vi "readslow.vi"(5 "Write enable":bool, 6 "Iteration number":i32, 7 "string":string, 8 "Slow data time":i32, 9 "mean value input":dbl[](array[numeric]), 10 "data  in":string[](array[string]), 11 "refnum in":refnum<file>) -> (0 "error out":errorcluster, 1 "mean value output":dbl[](array[numeric]), 2 "data out":string[](array[string]), 3 "refnum out":refnum<file>, 4 "Number of errors":bool)   [LabVIEW 2012]
panel:
  in  "array of datanames":string[](array[string])
  in  "number of iterations to\nbuild mean value":i32=5
  out "slow data time":u64
  out "mean value":dbl[](array[numeric])
  out "array of datanames":string[](array[string])
  out "data":string[](array[string])
  in  "Write Enable":bool
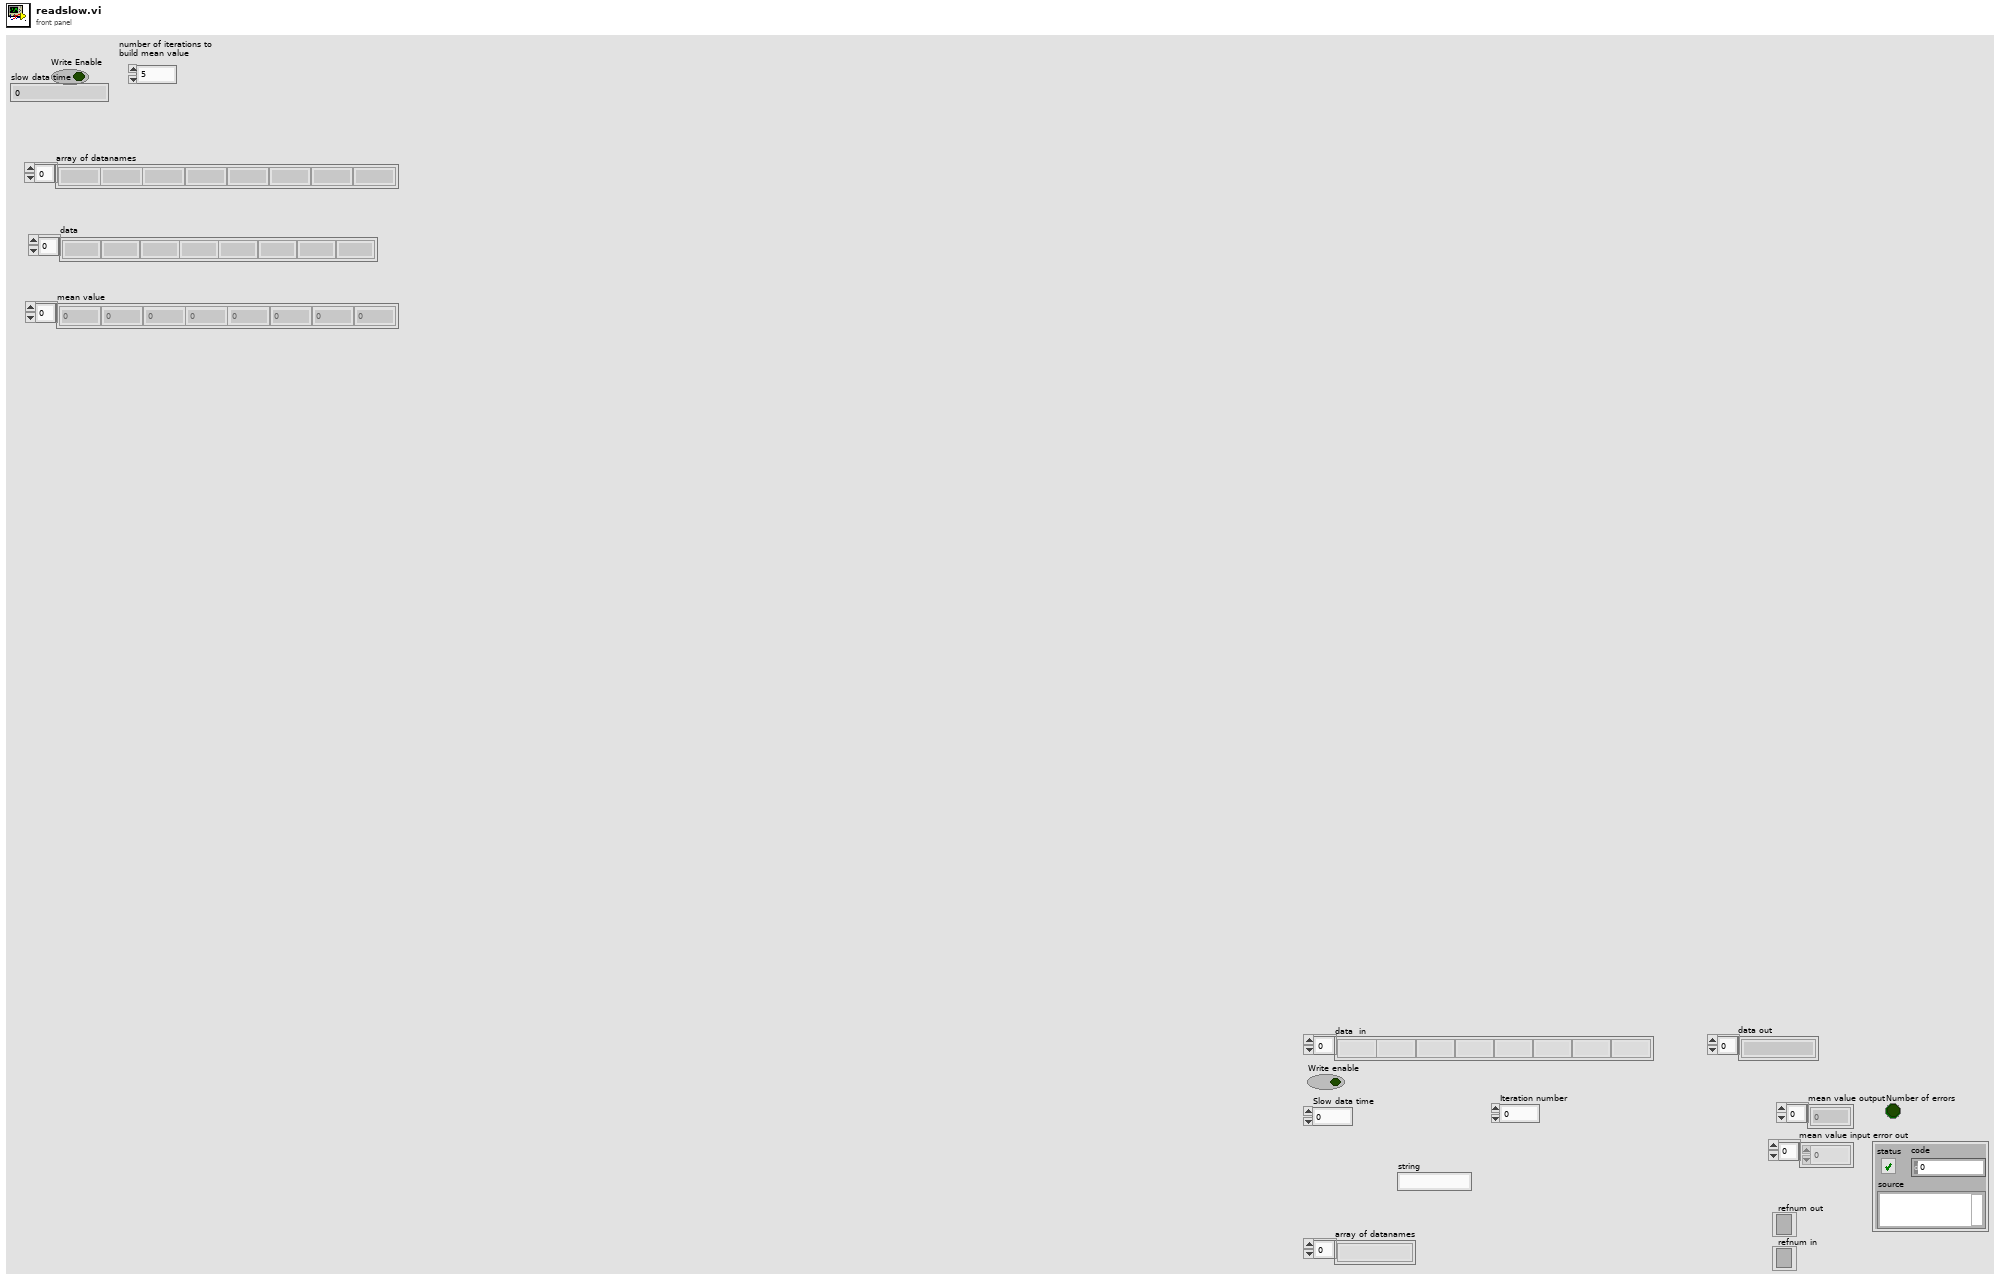
[diagram p1: front panel]
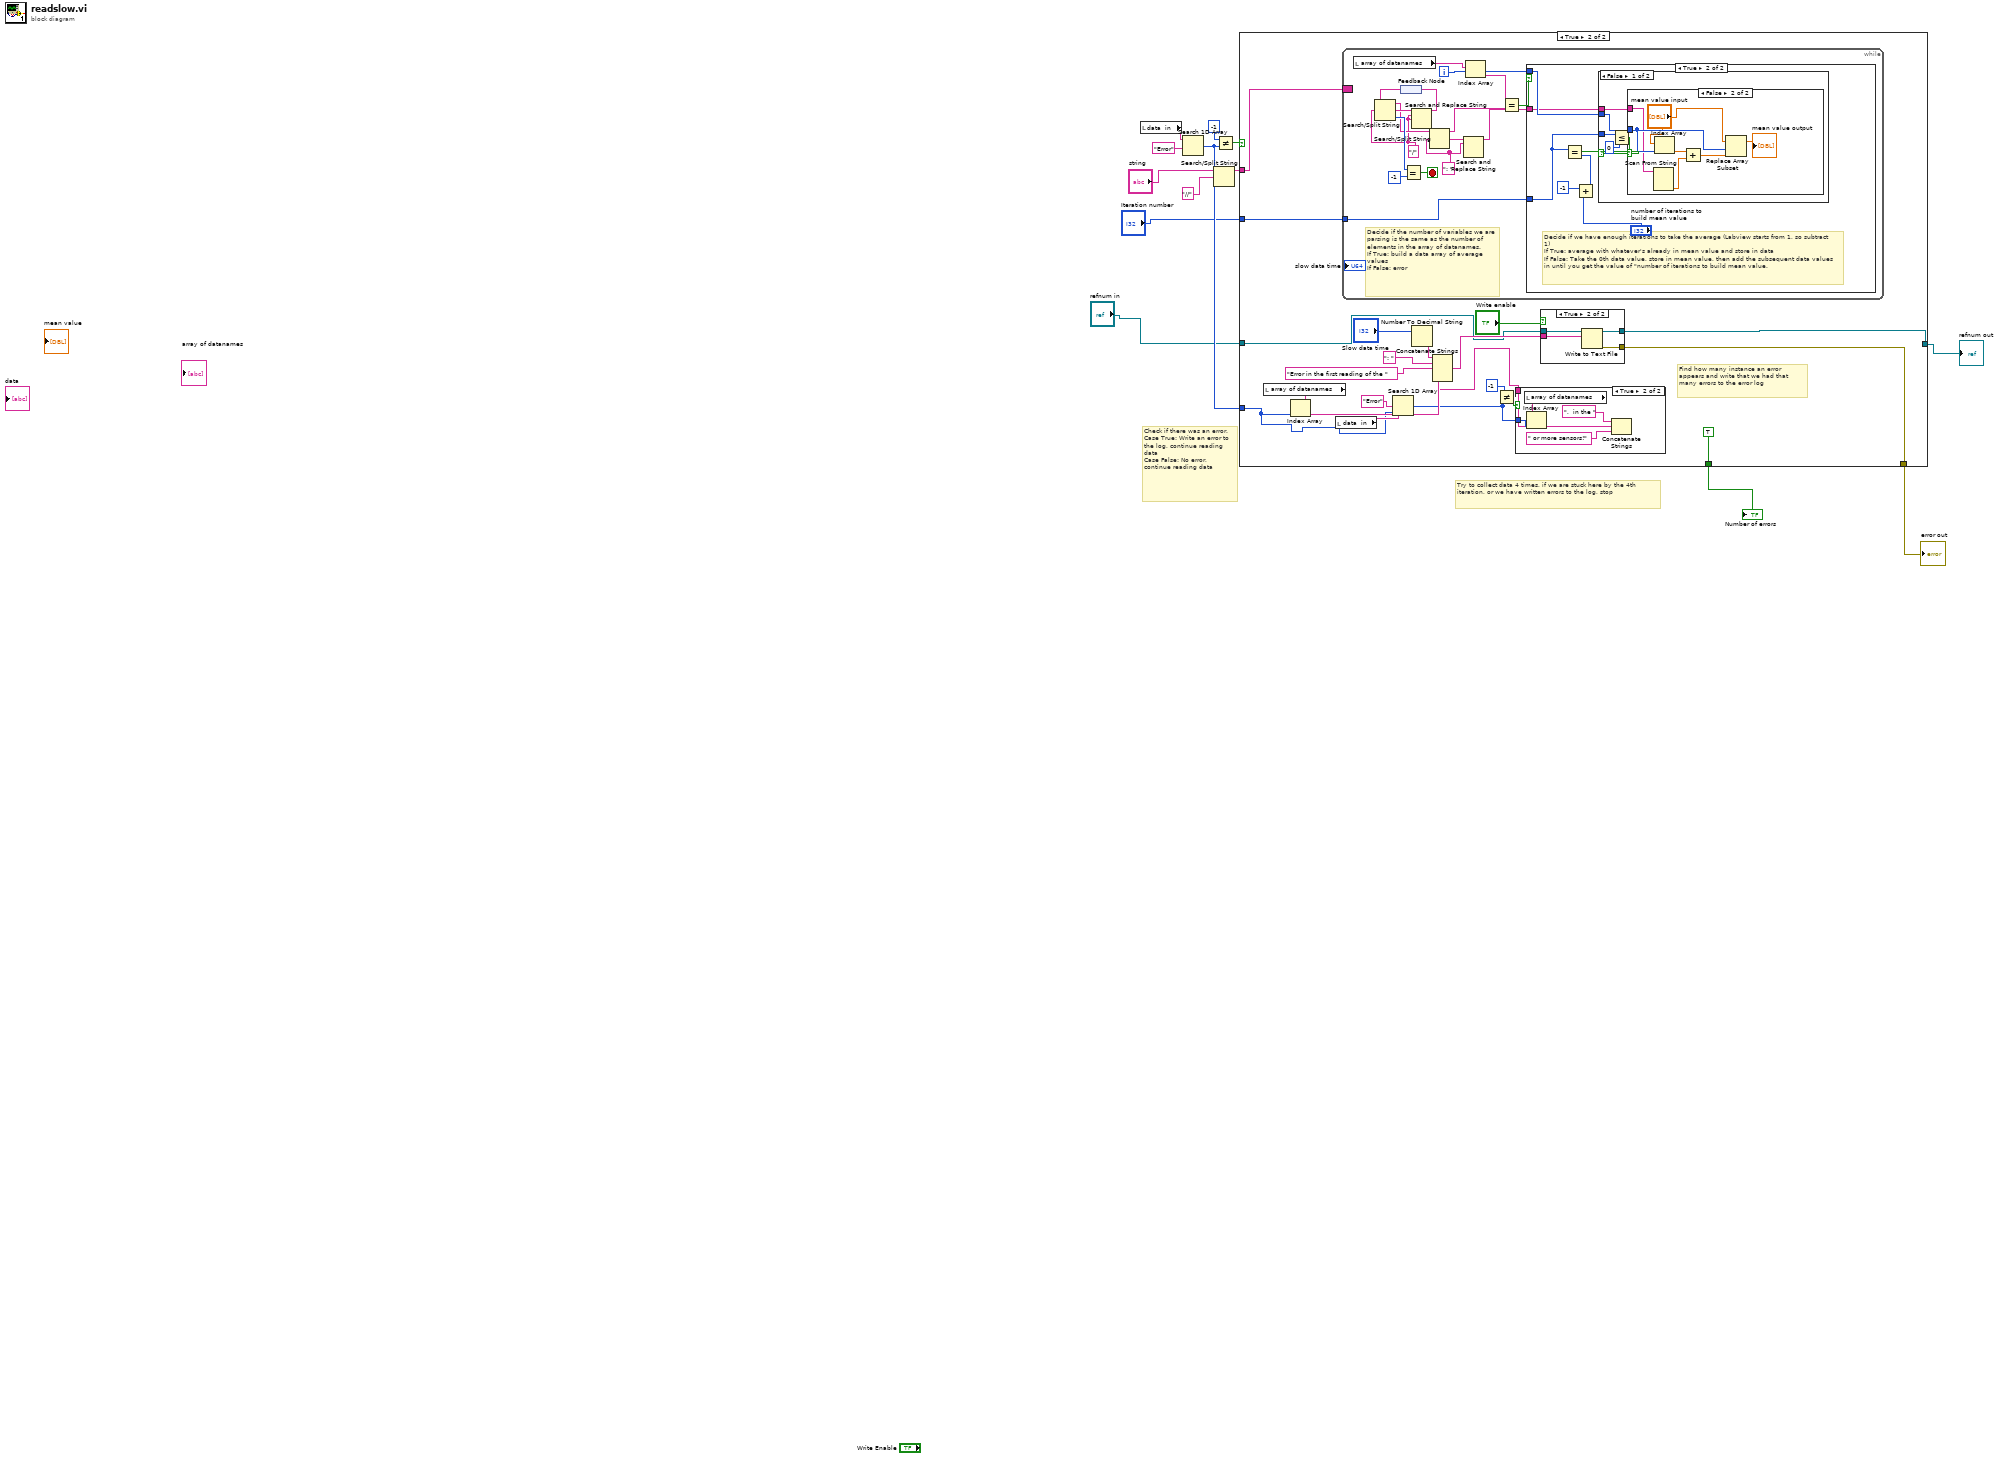
[diagram p0: block diagram]
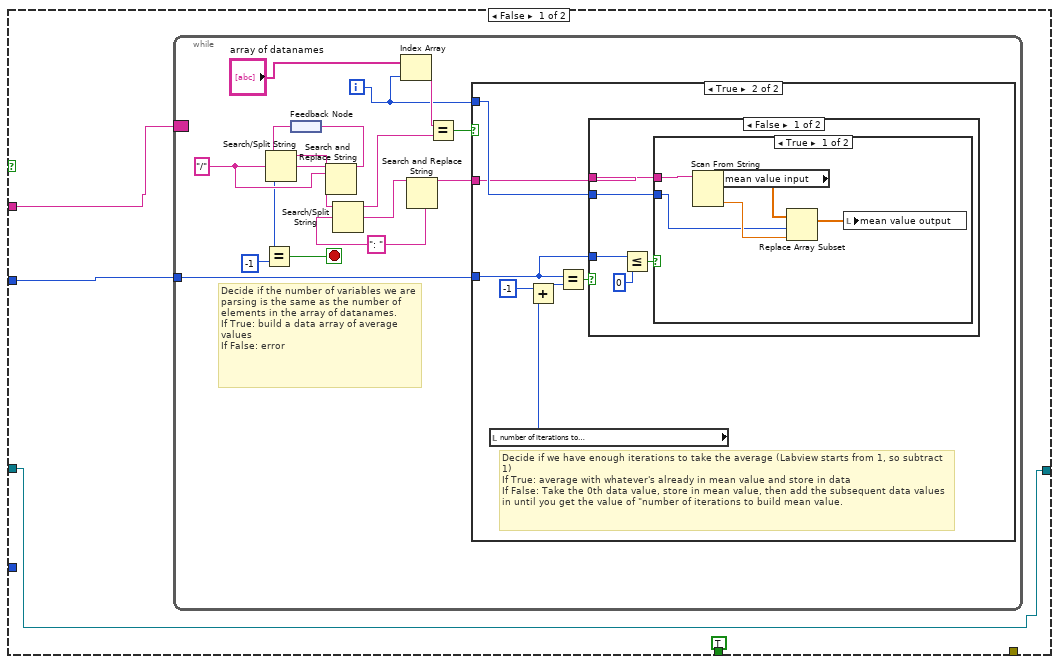
[diagram p2: hidden frame]
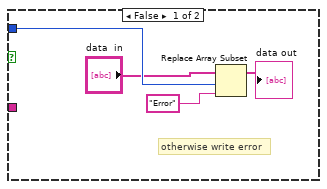
[diagram p3: hidden frame]
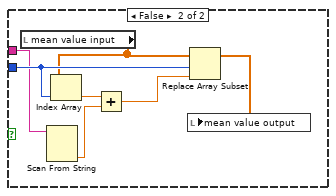
[diagram p4: hidden frame]
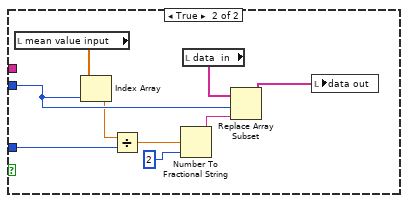
[diagram p5: hidden frame]
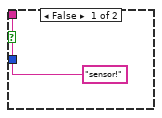
[diagram p7: hidden frame]
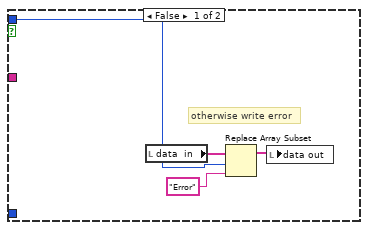
[diagram p8: hidden frame]
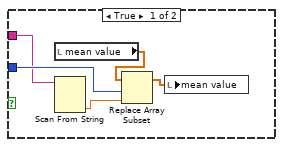
[diagram p9: hidden frame]
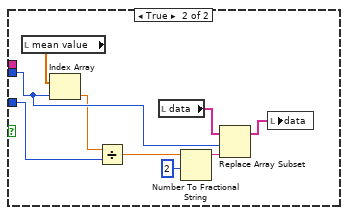
[diagram p10: hidden frame]
diagram:
  # "Try to collect data 4 times, if we are stuck here by the 4th iteration, or we have written errors to the log, stop"
  # "Check if there was an error.  \nCase True: Write an error to the log, continue reading data\nCase False: No error, continue reading data"
  n1 = local read "data  in"() -> (w9:string[])
  n2 = Search 1D Array(1D array=w9, element="Error") -> (index of element=w10:i32)  [unwired: 1 in]
  n3 = Search/Split String(string="string", search string/char (-)="//") -> (substring before match=w2:string)  [unwired: 1 in, 2 out]
  n4 = Not Equal?(x=-1 ("y"), y=w10) -> (x != y?=w8:bool)
  n5 = case shown="True" w8 {
    tunnel: w10 -> [_ w75]
    tunnel: [TRUE TRUE] -> w7
    tunnel: "refnum in" -> [w15 w79]
    tunnel: [_ w78] -> w12
    tunnel: "Iteration number" -> [w16 w77]
    tunnel: [w15 w76] -> w5
    tunnel: w2 -> [w14 w72]
    frame False {
      n6 = while {
        border: w14 -> [_]
        tunnel: w16 -> [w20]
        i -> [w19]
        stop <- w34 stop-if-true
        w23 = ": " ("format string")
        w29 = "/" ("search string/char (-)")
        # "Decide if the number of variables we are parsing is the same as the number of elements in the array of datanames.  \nIf True: build a data array of average values\nIf False: error"
        n7 = feedback #1() -> (w32:string)
        n8 = Search/Split String(string=w32, search string/char (-)=w29) -> (substring before match=w24:string, match + rest of string=w31:string, offset of match=w28:i32)  [unwired: 1 in]
        n9 = Equal?(x=w28, y=-1) -> (x = y?=w34:bool)
        n10 = Search and Replace String(input string=w31, search string=w29) -> (result string=w30:string)  [unwired: 6 in, 3 out]
        n11 = feedback-in #1(w30) -> ()
        n12 = Search/Split String(string=w24, search string/char (-)=w23) -> (substring before match=w27:string, match + rest of string=w25:string)  [unwired: 1 in, 1 out]
        n13 = Index Array(array="array of datanames", index=w19) -> (element=w26:string)
        n14 = Search and Replace String(input string=w25, search string=w23) -> (result string=w21:string)  [unwired: 6 in, 3 out]
        n15 = Equal?(x=w26, y=w27) -> (x = y?=w22:bool)
        n16 = case shown="True" w22 {
          tunnel: w21 -> [_ w44]
          tunnel: w19 -> [w38 w45]
          tunnel: w20 -> [_ w42]
          frame False {
            # "otherwise write error"
            n17 = Replace Array Subset(array="data  in", new element="Error" ("new element/subarray"), index=w38) -> (→"data out":string[])
          }
          frame True {
            # "Decide if we have enough iterations to take the average (Labview starts from 1, so subtract 1)\nIf True: average with whatever's already in mean value and store in data\nIf False: Take the 0th data value, store in mean value, then add the subsequent data values in until you get the value of \"number of iterations to build mean value."
            n18 = local read "number of iterations to\nbuild mean value"() -> (w41:i32)
            n19 = Add(x=-1, y=w41) -> (x+y=w40:i32)
            n20 = Equal?(x=w42, y=w40) -> (x = y?=w43:bool)
            n21 = case shown="False" w43 {
              tunnel: w42 -> [w50 w67]
              tunnel: w45 -> [w47 w70]
              tunnel: w44 -> [w46 _]
              frame False {
                n22 = Less Or Equal?(x=w50, y=0) -> (x <= y?=w49:bool)
                n23 = case shown="True" w49 {
                  tunnel: w47 -> [w51 w61]
                  tunnel: w46 -> [w55 w60]
                  frame True {
                    n24 = Scan From String(input string=w55) -> (output 1=w54:dbl)  [unwired: 4 in, 3 out]
                    n25 = local read "mean value input"() -> (w53:dbl[])
                    n26 = Replace Array Subset(array=w53, new element=w54, index=w51) -> (w52:dbl[])
                    n27 = local write "mean value output"(w52) -> ()
                  }
                  frame False {
                    n28 = local read "mean value input"() -> (w56:dbl[])
                    n29 = Scan From String(input string=w60) -> (output 1=w59:dbl)  [unwired: 4 in, 3 out]
                    n30 = Index Array(array=w56, index=w61) -> (element=w57:dbl)
                    n31 = Add(x=w57, y=w59) -> (x+y=w58:dbl)
                    n32 = Replace Array Subset(array=w56, new element=w58, index=w61) -> (w62:dbl[])
                    n33 = local write "mean value output"(w62) -> ()
                  }
                }
              }
              frame True {
                n34 = local read "mean value input"() -> (w64:dbl[])
                n35 = Index Array(array=w64, index=w70) -> (element=w63:dbl)
                n36 = Divide(x=w63, y=w67) -> (x/y=w68:dbl)
                n37 = Number To Fractional String(number=w68, precision (6)=i16 2) -> (F-format string=w71:string)  [unwired: 2 in]
                n38 = local read "data  in"() -> (w69:string[])
                n39 = Replace Array Subset(array=w69, new element=w71, index=w70) -> (w66:string[])
                n40 = local write "data out"(w66) -> ()
              }
            }
          }
        }
      }
    }
    frame True {
      # "Find how many instance an error appears and write that we had that many errors to the error log"
      n41 = local read "array of datanames"() -> (w89:string[])
      n42 = Index Array(array=w89, index=w75) -> (element=w88:string)
      n43 = local read "data  in"() -> (w87:string[])
      n44 = while {
        border: w72 -> [_]
        tunnel: w77 -> [w107]
        i -> [w105]
        stop <- w121 stop-if-true
        w108 = ": " ("format string")
        w106 = "/" ("search string/char (-)")
        # "Decide if the number of variables we are parsing is the same as the number of elements in the array of datanames.  \nIf True: build a data array of average values\nIf False: error"
        n45 = local read "array of datanames"() -> (w111:string[])
        n46 = feedback #2() -> (w119:string)
        n47 = Search/Split String(string=w119, search string/char (-)=w106) -> (substring before match=w109:string, match + rest of string=w118:string, offset of match=w116:i32)  [unwired: 1 in]
        n48 = Equal?(x=w116, y=-1) -> (x = y?=w121:bool)
        n49 = Search and Replace String(input string=w118, search string=w106, replace string=w106) -> (result string=w117:string)  [unwired: 5 in, 3 out]
        n50 = feedback-in #2(w117) -> ()
        n51 = Search/Split String(string=w109, search string/char (-)=w108) -> (substring before match=w114:string, match + rest of string=w110:string)  [unwired: 1 in, 1 out]
        n52 = Search and Replace String(input string=w110, search string=w108) -> (result string=w115:string)  [unwired: 6 in, 3 out]
        n53 = Index Array(array=w111, index=w105) -> (element=w113:string)
        n54 = Equal?(x=w113, y=w114) -> (x = y?=w112:bool)
        n55 = case shown="True" w112 {
          tunnel: w115 -> [_ w131]
          tunnel: w105 -> [w125 w132]
          tunnel: w107 -> [_ w129]
          frame False {
            # "otherwise write error"
            n56 = local read "data  in"() -> (w124:string[])
            n57 = Replace Array Subset(array=w124, new element="Error" ("new element/subarray"), index=w125) -> (w123:string[])
            n58 = local write "data out"(w123) -> ()
          }
          frame True {
            # "Decide if we have enough iterations to take the average (Labview starts from 1, so subtract 1)\nIf True: average with whatever's already in mean value and store in data\nIf False: Take the 0th data value, store in mean value, then add the subsequent data values in until you get the value of \"number of iterations to build mean value."
            n59 = Add(x=-1, y="number of iterations to\nbuild mean value") -> (x+y=w128:i32)
            n60 = Equal?(x=w129, y=w128) -> (x = y?=w130:bool)
            n61 = case shown="False" w130 {
              tunnel: w129 -> [w137 w156]
              tunnel: w132 -> [w134 w158]
              tunnel: w131 -> [w133 _]
              frame False {
                n62 = Less Or Equal?(x=w137, y=0) -> (x <= y?=w136:bool)
                n63 = case shown="False" w136 {
                  tunnel: w134 -> [w139 w149]
                  tunnel: w133 -> [w138 w148]
                  frame True {
                    n64 = local read "mean value"() -> (w141:dbl[])
                    n65 = Scan From String(input string=w138) -> (output 1=w142:dbl)  [unwired: 4 in, 3 out]
                    n66 = Replace Array Subset(array=w141, new element=w142, index=w139) -> (w140:dbl[])
                    n67 = local write "mean value"(w140) -> ()
                  }
                  frame False {
                    n68 = Scan From String(input string=w148) -> (output 1=w147:dbl)  [unwired: 4 in, 3 out]
                    n69 = Index Array(array="mean value input", index=w149) -> (element=w146:dbl)
                    n70 = Add(x=w146, y=w147) -> (x+y=w145:dbl)
                    n71 = Replace Array Subset(array="mean value input", new element=w145, index=w149) -> (→"mean value output":dbl[])
                  }
                }
              }
              frame True {
                n72 = local read "mean value"() -> (w150:dbl[])
                n73 = Index Array(array=w150, index=w158) -> (element=w152:dbl)
                n74 = Divide(x=w152, y=w156) -> (x/y=w151:dbl)
                n75 = local read "data"() -> (w157:string[])
                n76 = Number To Fractional String(number=w151, precision (6)=i16 2) -> (F-format string=w154:string)  [unwired: 2 in]
                n77 = Replace Array Subset(array=w157, new element=w154, index=w158) -> (w155:string[])
                n78 = local write "data"(w155) -> ()
              }
            }
          }
        }
      }
      n79 = Search 1D Array(1D array=w87, element="Error", start index (0)=w75) -> (index of element=w83:i32)
      n80 = Number To Decimal String(number="Slow data time") -> (decimal integer string=w92:string)  [unwired: 1 in]
      n81 = Not Equal?(x=-1 ("y"), y=w83) -> (x != y?=w85:bool)
      n82 = case shown="True" w85 {
        tunnel: w83 -> [_ w103]
        tunnel: ["sensor!" w99] -> w82
        frame False {
        }
        frame True {
          n83 = local read "array of datanames"() -> (w104:string[])
          n84 = Index Array(array=w104, index=w103) -> (element=w101:string)
          n85 = Concatenate Strings(",  in the " ("string"), w101, " or more sensors!" ("string")) -> (w99:string)
        }
      }
      n86 = Concatenate Strings(w92, ": ", "Error in the first reading of the ", w88, w82) -> (w81:string)
      n87 = case shown="True" "Write enable" {
        tunnel: w81 -> [_ w97]
        tunnel: w79 -> [w93 w94]
        tunnel: [_ w96] -> w78
        tunnel: [w93 w95] -> w76
        frame False {
        }
        frame True {
          n88 = Write to Text File(file (use dialog)=w94, text=w97) -> (refnum out=w95:refnum<file>, error out=w96:errorcluster)  [unwired: 2 in, 1 out]
        }
      }
    }
  }
  "error out" <- w12
  "Number of errors" <- w7
  "refnum out" <- w5
